vi "Bloomy BS120x Operational Example.vi"() -> ()   [LabVIEW 2021]
uses:
  src/TypeDefs/System Status.ctl
  src/TypeDefs/UnitType.ctl
  src/Public/New BS120x Device/New BS120x Ethernet Device.vi
  src/Public/New BS120x Device/New BS120x XNET Device.vi
  src/BS120x.lvclass
  src/BS120x Driver.lvlib
panel:
  out "error out":errorcluster
  in  "Channel":u16(ring) items=["All", "1", "2", "3", "4", "5", "6", "7", "8", "9", "10", "11", "12"]
  in  "Unit Type":T1=enum."BS1201"
  in  "Precision":bool
  in  "PID Disable":bool
  in  "DIO Direction":bool[](array[boolean])
  in  "DIO Control State":bool[](array[boolean])
  out "DIO Readback":bool[](array[boolean])
  out "Analog Input Readback":dbl[](array[numeric])
  out "Cell Current":dbl[](array[numeric]) format="%#8.1f"
  out "Cell Voltages":dbl[](array[numeric])
  in  "AO1 Voltage":dbl
  in  "AO2 Voltage":dbl
  in  "State":bool
  in  "Sink \nCurrent":dbl
  in  "Source \nCurrent":dbl
  out "Status":T2
  in  "Voltage":dbl=5.0 min=0.0 max=5.0 step=0.5
  in  "stop":bool
  in  "Protocol":enum32{"Ethernet", "XNET"}(tab)
  in  "Box IP address":string="192.168.1.101"
  in  "TCP port":u16=12345
  in  "UDP port":u16=54321
  in  "Reset Unit":bool
  in  "Box IDs":u8[](array[numeric])=[1]
  in  "CAN Interface":refnum<k21>
  in  "Current Box ID":u8
  # "Initialization & Configuration"
  # "Cell Control & Readback"
  # "Readback Data"
  # "Control Outputs"
  # "1"
  # "V"
  # "6"
  # "Operational Config\n(BS1201 Only)"
  # "mA"
  # "mA"
  # "12"
  # "Auxiliary Analog IO"
  # "Auxiliary Digital IO"
  # "1"
  # "4"
  # "8"
  # "(c) 2024 Bloomy Controls, Inc. All rights reserved."
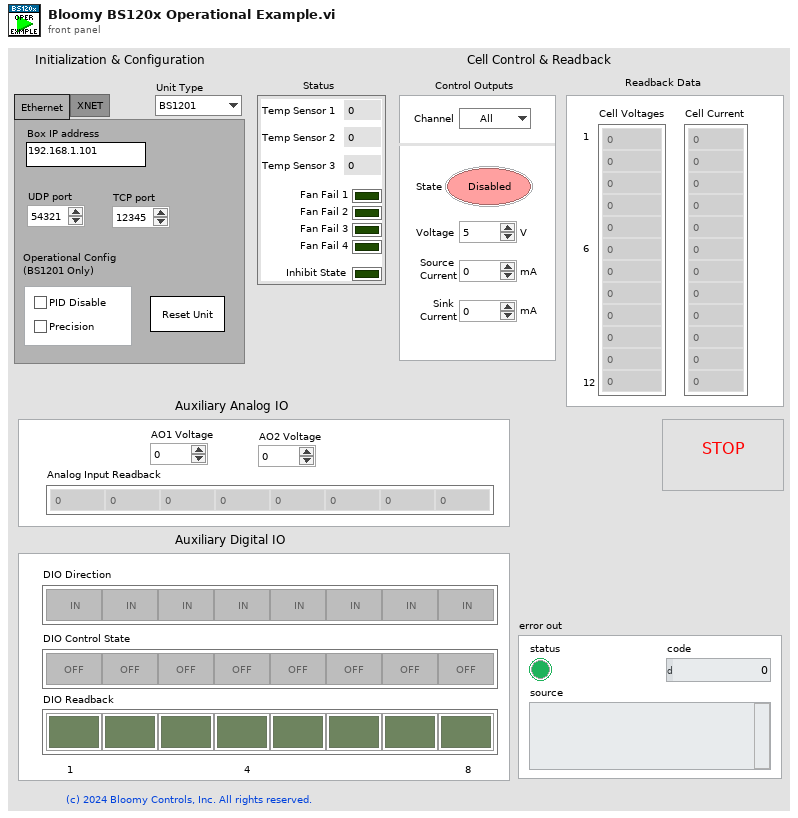
[diagram p1: front panel]
types:
  T1 = typedef "BS120x Driver.lvlib/BS120x.lvclass/UnitType.ctl" = enum16{"BS1200", "BS1201"}
  T2 = typedef "BS120x Driver.lvlib/BS120x.lvclass/System Status.ctl" = cluster{"Temp Sensor 1":dbl, "Temp Sensor 2":dbl, "Temp Sensor 3":dbl, "Fan Fail 1":bool, "Fan Fail 2":bool, "Fan Fail 3":bool, "Fan Fail 4":bool, "Inhibit State":bool}
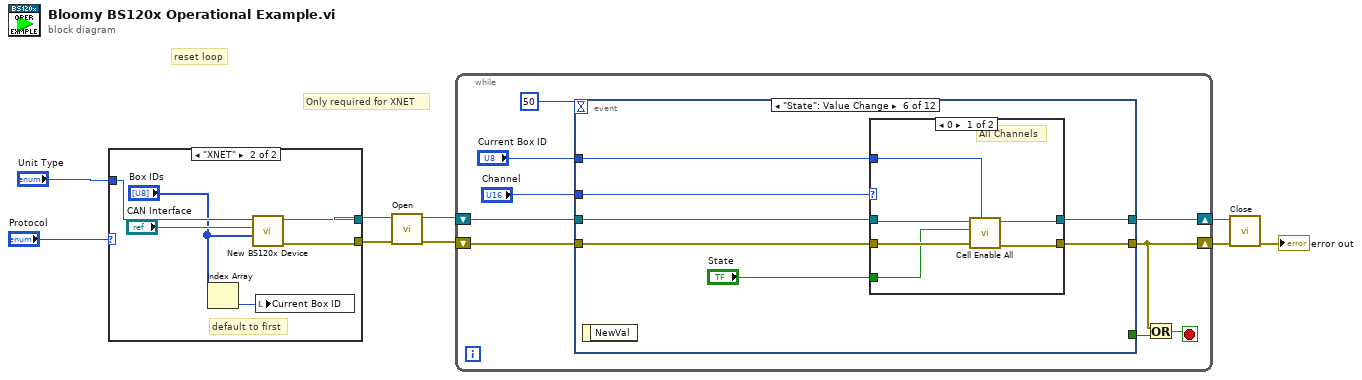
[diagram p0: block diagram]
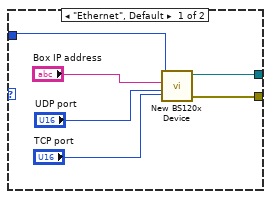
[diagram p2: hidden frame]
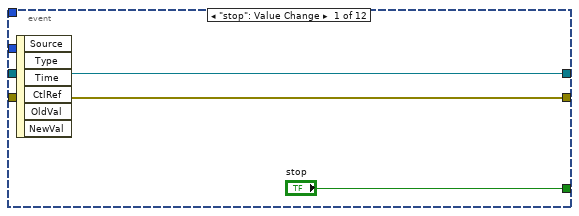
[diagram p3: hidden frame]
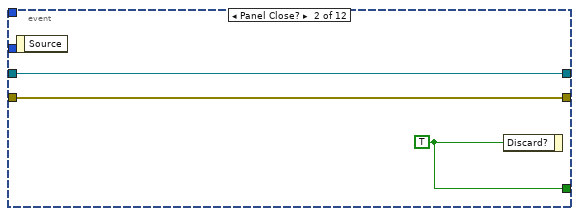
[diagram p4: hidden frame]
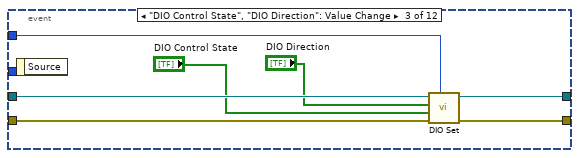
[diagram p5: hidden frame]
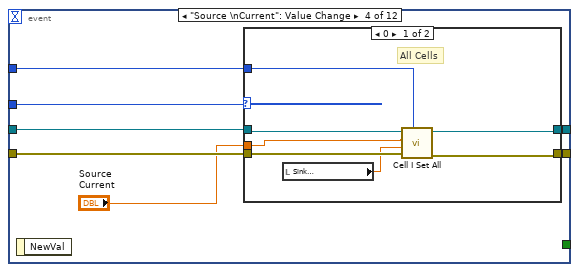
[diagram p6: hidden frame]
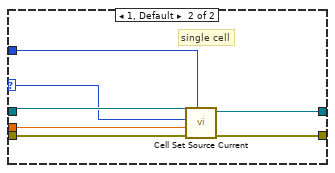
[diagram p7: hidden frame]
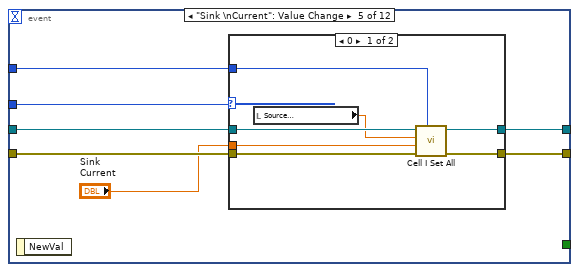
[diagram p8: hidden frame]
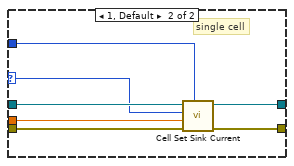
[diagram p9: hidden frame]
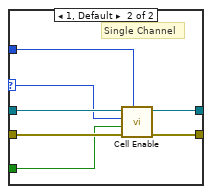
[diagram p10: hidden frame]
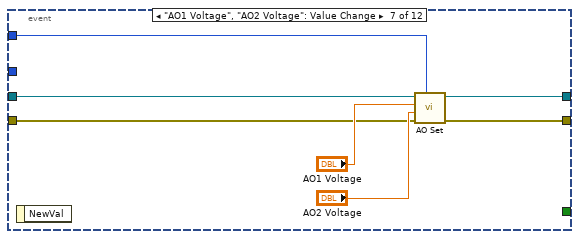
[diagram p11: hidden frame]
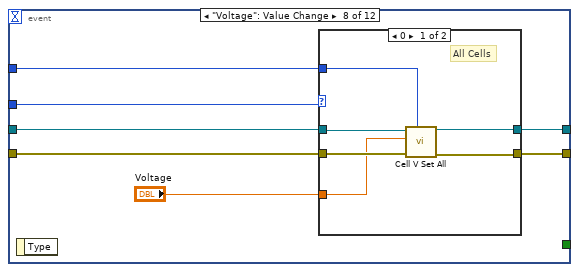
[diagram p12: hidden frame]
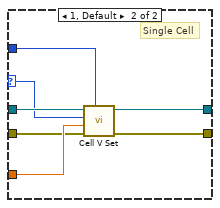
[diagram p13: hidden frame]
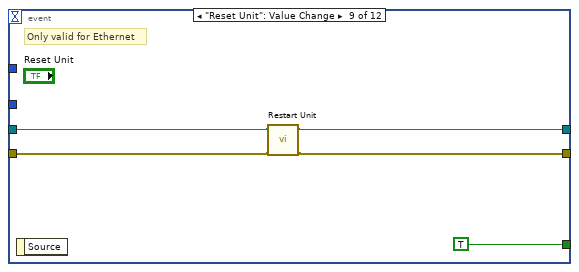
[diagram p14: hidden frame]
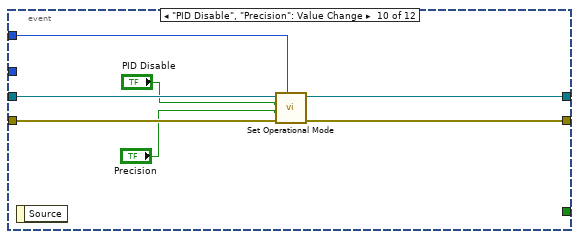
[diagram p15: hidden frame]
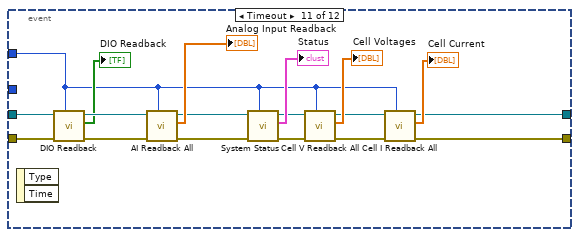
[diagram p16: hidden frame]
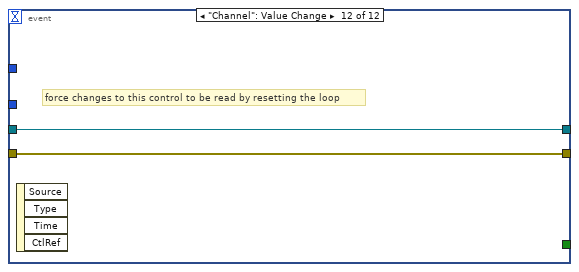
[diagram p17: hidden frame]
diagram:
  # "Only required for XNET"
  # "reset loop"
  n1 = case shown="\"XNET\"" "Protocol" {
    tunnel: "Unit Type" -> [w12 w19]
    tunnel: [w11 w21] -> w6
    tunnel: [w10 w20] -> w4
    frame "Ethernet", Default {
      n2 = call-poly "New BS120x Device.vi"("TCP port"="TCP port", "UDP port"="UDP port", "Box IP address"="Box IP address", "Unit Type"=w12) -> ("error out"=w10:errorcluster, "BS120x Out"=w11:refnum<class "BS120x.lvclass">)  [unwired: 6 in]
    }
    frame "XNET" {
      # "default to first"
      n3 = Index Array(array="Box IDs") -> (element=w16:u8)  [unwired: 1 in]
      n4 = call-poly "New BS120x Device.vi"("Box IDs"="Box IDs", "CAN Interface"="CAN Interface", "Unit Type"=w19) -> ("error out"=w20:errorcluster, "BS120x out"=w21:refnum<class "BS120x.lvclass">)  [unwired: 7 in]
      n5 = local write "Current Box ID"(w16) -> ()
    }
  }
  n6 = call-dynamic "Open.vi"("error in (no error)"=w4, "BS120x in"=w6) -> ("error out"=w3:errorcluster, "BS120x out"=w5:refnum<class "BS120x.lvclass">)  [unwired: 8 in]
  n7 = while {
    shift-right: [w24] -> w9
    shift-left: w3 -> [w28]
    shift-right: [w30] -> w8
    shift-left: w5 -> [w29]
    stop <- w26 stop-if-true
    n8 = event shown="[5] \"State\": Value Change" {
      selector: _ -> [_ _ _ _ _ _ _ _ _ _ _ _]
      dyn-events: _ -> [_ _ _ _ _ _ _ _ _ _ _ _]
      timeout: 50 -> [_ _ _ _ _ _ _ _ _ _ _ _]
      tunnel: [w33 w36 w39 w47 w68 w90 w108 w115 w134 w141 w159 w164] -> w30
      tunnel: w29 -> [w33 w36 w43 w50 w71 w91 w107 w118 w133 w142 w150 w164]
      tunnel: [w32 w34 w38 w48 w67 w89 w109 w116 w135 w143 w157 w163] -> w24
      tunnel: w28 -> [w32 w34 w40 w49 w70 w92 w110 w117 w136 w144 w149 w163]
      tunnel: ["stop" w35 _ _ _ _ _ _ TRUE ("Discard?") _ _ _] -> w25
      tunnel: "Channel" -> [_ _ _ w45 w66 w87 _ w114 _ _ _ _]
      tunnel: "Current Box ID" -> [_ _ w37 w44 w65 w86 w106 w113 _ w138 w145 _]
      event "stop": Value Change {
        n9 = event-data() -> ()  [unwired: 1 in, 6 out]
      }
      event Panel Close? {
        w35 = TRUE ("Discard?")
        n10 = event-data() -> ()  [unwired: 1 in, 1 out]
        n11 = event-data("Discard?"=w35) -> ()  [unwired: 1 in, 1 out]
      }
      event "DIO Control State", "DIO Direction": Value Change {
        n12 = event-data() -> ()  [unwired: 1 in, 1 out]
        n13 = call-dynamic "DIO Set.vi"("Box ID"=w37, "error in (no error)"=w40, "DIO Enable"="DIO Control State", "DIO Direction"="DIO Direction", "BS120x in"=w43) -> ("error out"=w38:errorcluster, "BS120x out"=w39:refnum<class "BS120x.lvclass">)  [unwired: 5 in]
      }
      event "Source \nCurrent": Value Change {
        n14 = event-data() -> ()  [unwired: 1 in, 1 out]
        n15 = case shown="0" w45 {
          selector: w45 -> [_ w59]
          tunnel: w50 -> [w56 w64]
          tunnel: w49 -> [w55 w63]
          tunnel: [w54 w62] -> w48
          tunnel: [w57 w61] -> w47
          tunnel: "Source \nCurrent" -> [w53 w60]
          tunnel: w44 -> [w51 w58]
          frame 0 {
            # "All Cells"
            n16 = local read "Sink \nCurrent"() -> (w52:dbl)
            n17 = call-dynamic "Cell I Set All.vi"("Box ID"=w51, "error in (no error)"=w55, "Sink I All"=w52, "Source I All"=w53, "BS120x in"=w56) -> ("error out"=w54:errorcluster, "BS120x out"=w57:refnum<class "BS120x.lvclass">)  [unwired: 5 in]
          }
          frame 1, Default {
            # "single cell"
            n18 = call-dynamic "Cell Set Source Current.vi"("Box ID"=w58, "error in (no error)"=w63, "Source Current Limit (mA)"=w60, "Channel"=w59, "BS120x in"=w64) -> ("error out"=w62:errorcluster, "BS120x out"=w61:refnum<class "BS120x.lvclass">)  [unwired: 5 in]
          }
        }
      }
      event "Sink \nCurrent": Value Change {
        n19 = event-data() -> ()  [unwired: 1 in, 1 out]
        n20 = case shown="0" w66 {
          selector: w66 -> [_ w80]
          tunnel: w71 -> [w76 w85]
          tunnel: w70 -> [w75 w84]
          tunnel: "Sink \nCurrent" -> [w74 w83]
          tunnel: [w77 w82] -> w68
          tunnel: [w78 w81] -> w67
          tunnel: w65 -> [w72 w79]
          frame 0 {
            n21 = local read "Source \nCurrent"() -> (w73:dbl)
            n22 = call-dynamic "Cell I Set All.vi"("Box ID"=w72, "error in (no error)"=w75, "Sink I All"=w74, "Source I All"=w73, "BS120x in"=w76) -> ("error out"=w78:errorcluster, "BS120x out"=w77:refnum<class "BS120x.lvclass">)  [unwired: 5 in]
          }
          frame 1, Default {
            # "single cell"
            n23 = call-dynamic "Cell Set Sink Current.vi"("Box ID"=w79, "error in (no error)"=w84, "Sink Current Limit (mA)"=w83, "Channel"=w80, "BS120x in"=w85) -> ("error out"=w81:errorcluster, "BS120x out"=w82:refnum<class "BS120x.lvclass">)  [unwired: 5 in]
          }
        }
      }
      event "State": Value Change {
        n24 = event-data() -> ()  [unwired: 1 in, 1 out]
        n25 = case shown="0" w87 {
          selector: w87 -> [_ w100]
          tunnel: w92 -> [w97 w105]
          tunnel: w91 -> [w98 w104]
          tunnel: [w96 w103] -> w90
          tunnel: [w95 w102] -> w89
          tunnel: "State" -> [w94 w101]
          tunnel: w86 -> [w93 w99]
          frame 0 {
            # "All Channels"
            n26 = call-dynamic "Cell Enable All.vi"("Box ID"=w93, "error in (no error)"=w97, "Enable"=w94, "BS120x in"=w98) -> ("error out"=w95:errorcluster, "BS120x out"=w96:refnum<class "BS120x.lvclass">)  [unwired: 6 in]
          }
          frame 1, Default {
            # "Single Channel"
            n27 = call-dynamic "Cell Enable.vi"("Box ID"=w99, "error in (no error)"=w105, "Enable"=w101, "Channel"=w100, "BS120x in"=w104) -> ("error out"=w102:errorcluster, "BS120x out"=w103:refnum<class "BS120x.lvclass">)  [unwired: 5 in]
          }
        }
      }
      event "AO1 Voltage", "AO2 Voltage": Value Change {
        n28 = event-data() -> ()  [unwired: 1 in, 1 out]
        n29 = call-dynamic "AO Set.vi"("Box ID"=w106, "error in (no error)"=w110, "AO2 Voltage"="AO2 Voltage", "AO1 Voltage"="AO1 Voltage", "BS120x in"=w107) -> ("error out"=w109:errorcluster, "BS120x out"=w108:refnum<class "BS120x.lvclass">)  [unwired: 5 in]
      }
      event "Voltage": Value Change {
        n30 = event-data() -> ()  [unwired: 1 in, 1 out]
        n31 = case shown="0" w114 {
          selector: w114 -> [_ w127]
          tunnel: "Voltage" -> [w121 w132]
          tunnel: w118 -> [w125 w131]
          tunnel: w117 -> [w124 w130]
          tunnel: [w123 w129] -> w116
          tunnel: [w122 w128] -> w115
          tunnel: w113 -> [w120 w126]
          frame 0 {
            # "All Cells"
            n32 = call-dynamic "Cell V Set All.vi"("Box ID"=w120, "error in (no error)"=w124, "Voltage"=w121, "BS120x in"=w125) -> ("error out"=w123:errorcluster, "BS120x out"=w122:refnum<class "BS120x.lvclass">)  [unwired: 6 in]
          }
          frame 1, Default {
            # "Single Cell"
            n33 = call-dynamic "Cell V Set.vi"("Box ID"=w126, "error in (no error)"=w130, "Voltage"=w132, "Channel"=w127, "BS120x in"=w131) -> ("error out"=w129:errorcluster, "BS120x out"=w128:refnum<class "BS120x.lvclass">)  [unwired: 5 in]
          }
        }
      }
      event "Reset Unit": Value Change {
        # "Only valid for Ethernet"
        n34 = event-data() -> ()  [unwired: 1 in, 1 out]
        n35 = call-dynamic "Restart Unit.vi"("error in (no error)"=w136, "BS120x in"=w133) -> ("error out"=w135:errorcluster, "BS120x out"=w134:refnum<class "BS120x.lvclass">)  [unwired: 8 in]
      }
      event "PID Disable", "Precision": Value Change {
        n36 = event-data() -> ()  [unwired: 1 in, 1 out]
        n37 = call-dynamic "Set Operational Mode.vi"("Box ID"=w138, "error in (no error)"=w144, "Precision Mode"="Precision", "PID Disable"="PID Disable", "BS120x in"=w142) -> ("error out"=w143:errorcluster, "BS120x out"=w141:refnum<class "BS120x.lvclass">)  [unwired: 5 in]
      }
      event Timeout {
        n38 = event-data() -> ()  [unwired: 1 in, 2 out]
        n39 = call-dynamic "DIO Readback.vi"("Box ID"=w145, "error in (no error)"=w149, "BS120x in"=w150) -> ("error out"=w148:errorcluster, "DIO Readback"=→"DIO Readback":bool[], "BS120x out"=w147:refnum<class "BS120x.lvclass">)  [unwired: 6 in]
        n40 = call-dynamic "AI Readback All.vi"("Box ID"=w145, "error in (no error)"=w148, "BS120x in"=w147) -> ("error out"=w151:errorcluster, "Voltage"=→"Analog Input Readback":dbl[], "BS120x out"=w152:refnum<class "BS120x.lvclass">)  [unwired: 6 in]
        n41 = call-dynamic "System Status.vi"("Box ID"=w145, "error in (no error)"=w151, "BS120x in"=w152) -> ("error out"=w153:errorcluster, "Status"=→"Status":T2, "BS120x out"=w155:refnum<class "BS120x.lvclass">)  [unwired: 6 in]
        n42 = call-dynamic "Cell V Readback All.vi"("Box ID"=w145, "error in (no error)"=w153, "BS120x in"=w155) -> ("error out"=w154:errorcluster, "Voltage"=→"Cell Voltages":dbl[], "BS120x out"=w156:refnum<class "BS120x.lvclass">)  [unwired: 6 in]
        n43 = call-dynamic "Cell I Readback All.vi"("Box ID"=w145, "error in (no error)"=w154, "BS120x in"=w156) -> ("error out"=w157:errorcluster, "Current"=→"Cell Current":dbl[], "BS120x out"=w159:refnum<class "BS120x.lvclass">)  [unwired: 6 in]
      }
      event "Channel": Value Change {
        # "force changes to this control to be read by resetting the loop"
        n44 = event-data() -> ()  [unwired: 1 in, 4 out]
      }
    }
    n45 = Or(x=w24, y=w25) -> (x .or. y?=w26:bool)
  }
  n46 = call-dynamic "Close.vi"("error in (no error)"=w9, "BS120x In"=w8) -> ("error out"=→"error out":errorcluster)  [unwired: 8 in, 1 out]
